vi "Reset.vi"(8 "error in (no error)":errorcluster, 10 "Channel (0: SIM900)":i32(ring) items=["SIM900", "1", "2", "3", "4", "5", "6", "7", "8", "9", "A", "B", "C", "D"], 11 "VISA resource name":refnum<visa-resource-name>) -> (0 "error out":errorcluster, 3 "VISA resource name out":refnum<visa-resource-name>)   [LabVIEW 2019, in "Stanford Research SIM900 Series.lvlib"]
doc: "Resets the instrument and then sends a set of default setup commands to the instrument."
uses:
  Stanford Research SIM900 Series.lvlib
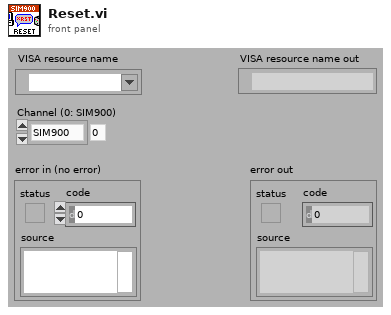
[diagram p1: front panel]
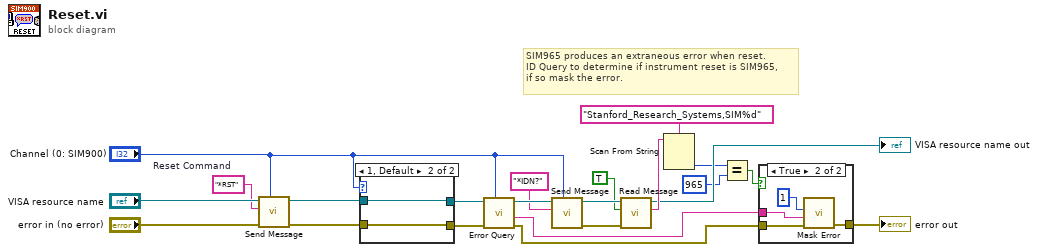
[diagram p0: block diagram]
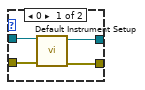
[diagram p3: hidden frame]
diagram:
  w16 = "*RST"  # Reset Command
  # "SIM965 produces an extraneous error when reset.\nID Query to determine if instrument reset is SIM965,\nif so mask the error."
  n1 = call "Send Message.vi"("Channel (0: SIM900)"="Channel (0: SIM900)", "error in (no error)"="error in (no error)", "Message (\"\")"=w16, "VISA resource name"="VISA resource name") -> ("error out"=w18:errorcluster, "VISA resource name out"=w20:refnum<visa-resource-name>)  [unwired: 6 in]
  n2 = case shown="1, Default" "Channel (0: SIM900)" {
    tunnel: [w26 w27] -> w22
    tunnel: [w25 w28] -> w21
    tunnel: w20 -> [w24 w28]
    tunnel: w18 -> [w23 w27]
    frame 0 {
      n3 = call "Default Instrument Setup.vi"("error in (no error)"=w23, "VISA resource name"=w24) -> ("error out"=w26:errorcluster, "VISA resource name out"=w25:refnum<visa-resource-name>)  [unwired: 8 in]
    }
    frame 1, Default {
    }
  }
  n4 = call "Error Query.vi"("Channel (0: SIM900)"="Channel (0: SIM900)", "error in (no error)"=w22, "VISA resource name"=w21) -> ("error out"=w1:errorcluster, "Error Message"=w12:string, "VISA resource name out"=w14:refnum<visa-resource-name>)  [unwired: 5 in, 1 out]
  n5 = call "Send Message.vi"("Channel (0: SIM900)"="Channel (0: SIM900)", "Message (\"\")"="*IDN?" ("Message (\"\")"), "VISA resource name"=w14) -> ("error out"=w2:errorcluster, "VISA resource name out"=w13:refnum<visa-resource-name>)  [unwired: 7 in]
  n6 = call "Read Message.vi"("error in (no error)"=w2, "Enable Header Information (False)"=TRUE ("From Port"), "VISA resource name"=w13) -> ("Message"=w8:string, "VISA resource name out"=→"VISA resource name out":refnum<visa-resource-name>)  [unwired: 6 in, 1 out]
  n7 = Scan From String(format string="Stanford_Research_Systems,SIM%d", input string=w8) -> (output 1=w5:i32)  [unwired: 3 in, 3 out]
  n8 = Equal?(x=w5, y=965) -> (x = y?=w3:bool)
  n9 = case shown="True" w3 {
    tunnel: w12 -> [_ w33]
    tunnel: [w29 w31] -> w15
    tunnel: w1 -> [w29 w30]
    frame False {
    }
    frame True {
      n10 = call "Mask Error.vi"("error in (no error)"=w30, "Error Message"=w33, "Error to Ignore"=1) -> ("error out"=w31:errorcluster)  [unwired: 8 in]
    }
  }
  "error out" <- w15
